vi "SrvSetCpuStatus.vi"(0 "ref in":u64, 7 "CpuStatus":i32(ring)=8 items=["Run"=8, "Stop"=4], 11 "error in (no error)":errorcluster) -> (4 "ref out":u64, 8 "return type":i32, 15 "error out":errorcluster)   [LabVIEW 2018, in "Snap7.lvlib"]
uses:
  Snap7.lvlib
  windows/lv_snap7.dll
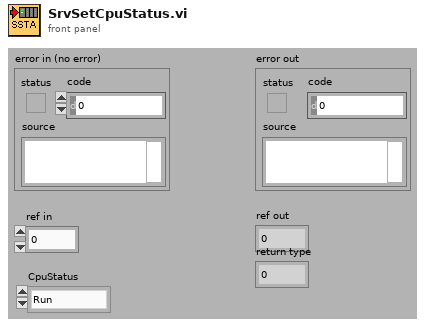
[diagram p1: front panel]
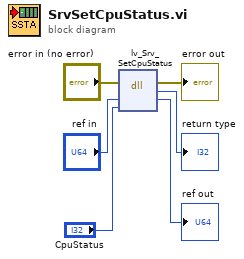
[diagram p0: block diagram]
diagram:
  n1 = dll-call lib="PTH2iabs D项目Feng恒隆项目Labview性能试验台SourcesSnap7libwindowslv_snap7.dll" fn="lv_Srv_SetCpuStatus"(error in="error in (no error)", "Server"="ref in", "Status"="CpuStatus") -> (error out=→"error out":errorcluster, "return type"=→"return type":i32, "Server"=→"ref out":u64)  [unwired: 3 in, 1 out]
